vi "call_opt_DispComp_matlab.vi"(8 "error in":errorcluster, 9 "Wavenumber":dbl[](array[numeric]), 10 "P":dbl[](array[numeric]), 11 "Raw image":u16[][](array[numeric])) -> (0 "error out":errorcluster, 1 "C3 out":dbl, 2 "C2 out":dbl, 3 "dispCompPhasor":cdb[](array[numeric]))   [LabVIEW 2017]
panel:
  out "debugging error":errorcluster
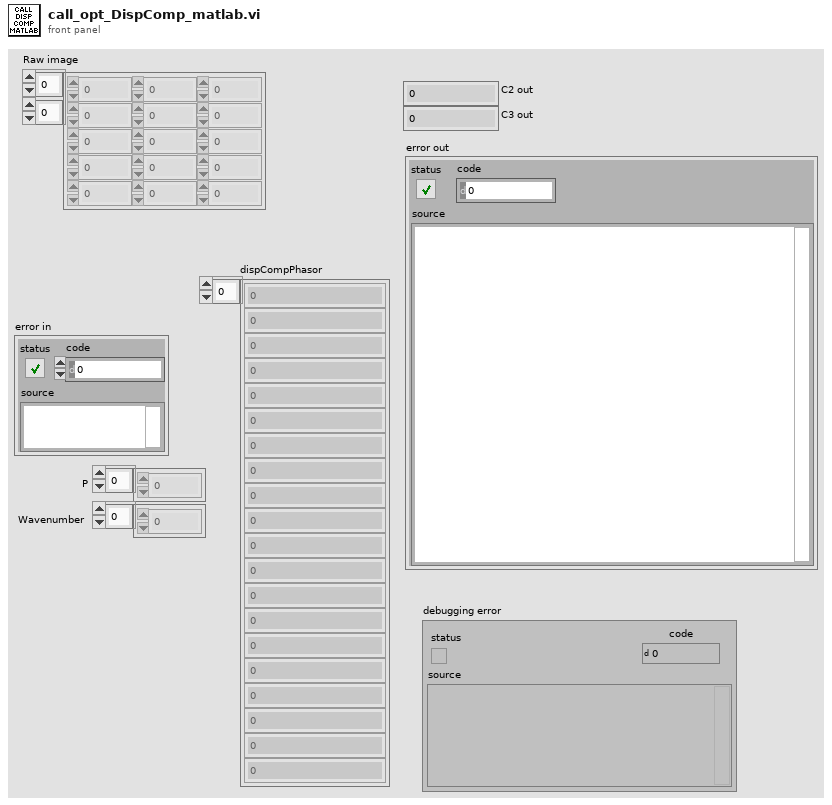
[diagram p1: front panel]
types:
  T1 = typedef "Image Type" = u32
  T2 = typedef "IMAQ Image.ctl" = refnum<image>
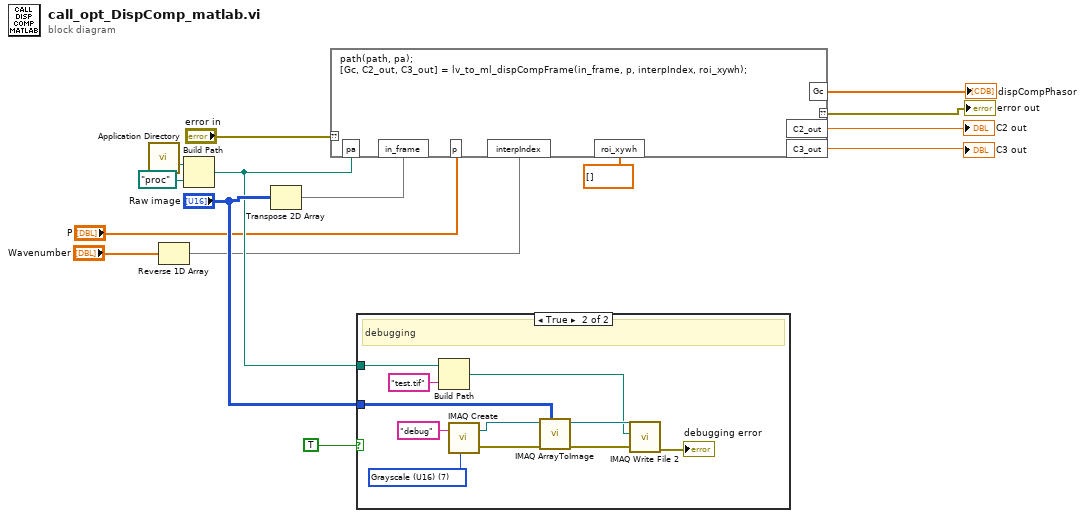
[diagram p0: block diagram]
diagram:
  n1 = call <vilib>:"Application Directory.vi"() -> ("Application Directory"=w15:path)
  n2 = Reverse 1D Array(array="Wavenumber") -> (reversed array=w1:dbl[])
  n3 = Build Path(base path=w15, name or relative path=path "proc") -> (appended path=w5:path)
  n4 = Transpose 2D Array(2D array="Raw image") -> (transposed array=w4:u16[][])
  n5 = script code="path(path, pa);\n[Gc, C2_out, C3_out] = lv_to_ml_dispCompFrame(in_frame, p, interpIndex, roi_xywh);"("??"="error in", "pa"=w5, "in_frame"=w4, "p"="P", "interpIndex"=w1, "roi_xywh"=dbl[] [] ("1-D Array of Real")) -> ("??"=→"error out":errorcluster, "C2_out"=→"C2 out":dbl, "C3_out"=→"C3 out":dbl, "Gc"=→"dispCompPhasor":cdb[])
  n6 = case shown="True" TRUE {
    tunnel: "Raw image" -> [_ w26]
    tunnel: w5 -> [_ w23]
    frame False {
    }
    frame True {
      w16 = T1 7 items=["Grayscale (U8)", "Grayscale (I16)", "Grayscale (SGL)", "Complex (CSG)", "RGB (U32)", "HSL (U32)", "RGB (U64)", "Grayscale (U16)"] ("Image Type")
      # "debugging"
      n7 = Build Path(base path=w23, name or relative path="test.tif") -> (appended path=w21:path)
      n8 = call "IMAQ Create"("Image Name"="debug", "Image Type"=w16) -> ("New Image"=w25:T2, "error out"=w20:errorcluster)  [unwired: 3 in]
      n9 = call "IMAQ ArrayToImage"("Image Pixels (U16)"=w26, "error in (no error)"=w20, "Image"=w25) -> ("error out"=w19:errorcluster, "Image Out"=w24:T2)  [unwired: 7 in]
      n10 = call-poly "IMAQ Write File 2"("error in (no error)"=w19, "File Path"=w21, "Image"=w24) -> ("error out"=→"debugging error":errorcluster)  [unwired: 7 in, 1 out]
    }
  }
